vi "RW Find Edge ROI.vi"(7 "Read/Write":enum16{"Read", "Write"}(ring), 8 "error in (no error)":errorcluster, 11 "Inspec part":T1) -> (0 "error out":errorcluster)   [LabVIEW 2017]
uses:
  Use Module/Algorithm Loop/Gentex Algo/inspec part.ctl
  File/Control/Parent path.ctl
  Toolbox/Control/CVT Action.ctl
  Toolbox/Control/CVT name.vi
  Section and key name.vi
  <vilib>/Utility/config.llb/Write Key (I32).vi
  <vilib>/Utility/config.llb/Write Key (Double).vi
  <vilib>/Utility/config.llb/Read Key (I32).vi
  <vilib>/Utility/config.llb/Read Key (Double).vi
  File/File.lvlib
  <vilib>/Utility/config.llb/NI_LVConfig.lvlib
  Toolbox/Toolbox.lvlib
  Use Module/Algorithm Loop/Algorithm API.lvlib
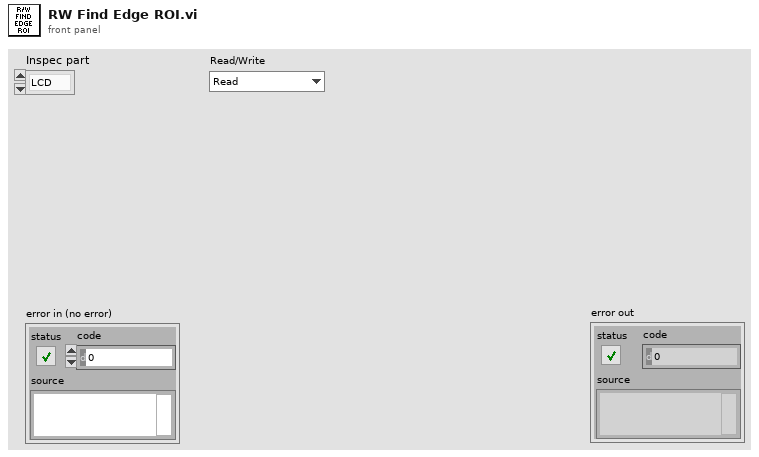
[diagram p1: front panel]
types:
  T1 = typedef "Algorithm API.lvlib/inspec part.ctl" = enum16{"LCD", "Housing"}
  T2 = typedef "File.lvlib/Parent path.ctl" = enum16{"Project", "Setting", "Log"}
  T3 = typedef "Toolbox.lvlib/CVT Action.ctl" = enum16{"Set", "Replace", "Get", "Check", "Delete", "Delete All"}
  T4 = typedef "ROI Descriptor" = cluster{"Global Rectangle":i32[], "Contours":cluster{"ID":enum32{"External", "Internal"}, "Type":u32, "Coordinates":i32[]}[]}
  T5 = typedef "IMAQ Rectangle" = cluster{"Left":i32, "Top":i32, "Right":i32, "Bottom":i32, "Rotation":dbl}
  T6 = typedef "NI_LVConfig.lvlib/Config Data RefNum.ctl" = refnum<k1>
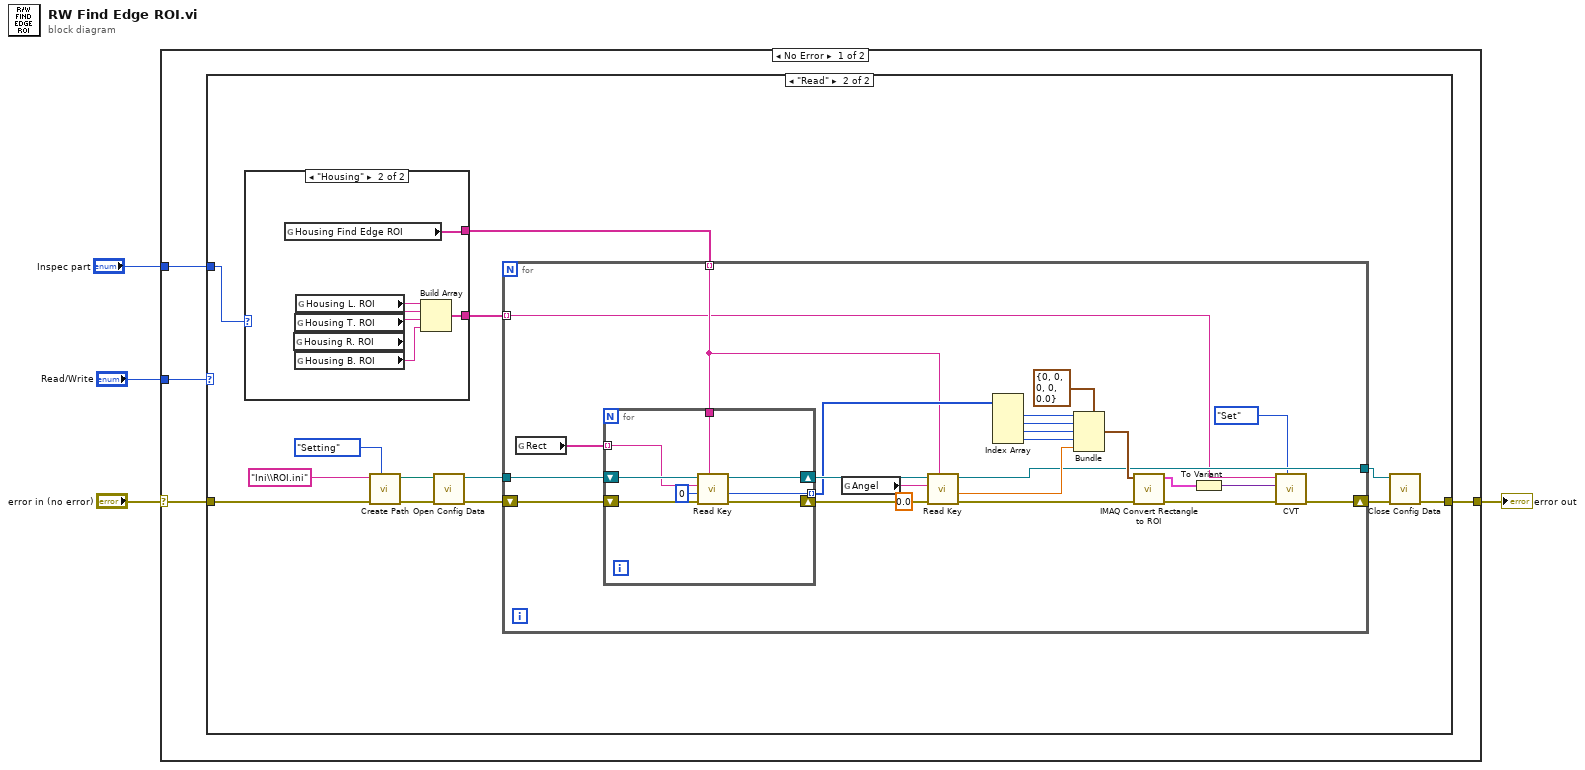
[diagram p0: block diagram]
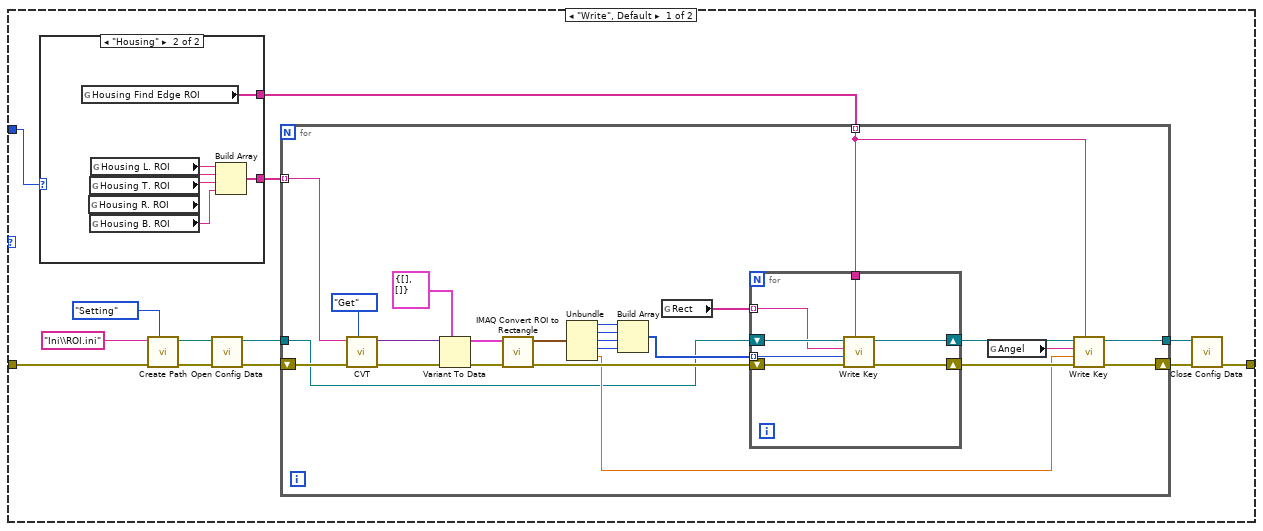
[diagram p2: hidden frame]
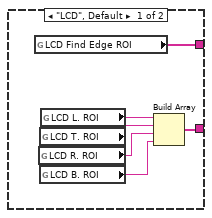
[diagram p3: hidden frame]
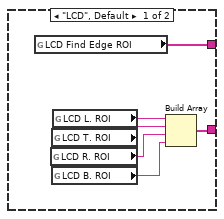
[diagram p4: hidden frame]
diagram:
  n1 = case shown="No Error" "error in (no error)" {
    selector: "error in (no error)" -> [w8 w122]
    tunnel: [w7 w122] -> w3
    tunnel: "Read/Write" -> [w6 _]
    tunnel: "Inspec part" -> [w5 _]
    frame No Error {
      n2 = case shown="\"Read\"" w6 {
        tunnel: w8 -> [w21 w77]
        tunnel: [w14 w70] -> w7
        tunnel: w5 -> [w10 w66]
        frame "Write", Default {
          n3 = case shown="\"Housing\"" w10 {
            tunnel: [w23 w29] -> w11
            tunnel: [w22 w28] -> w9
            frame "LCD", Default {
              n4 = global read "Section and key name.vi" "LCD Find Edge ROI"() -> (w22:string[])
              n5 = global read "CVT name.vi" "LCD R. ROI"() -> (w25:string)
              n6 = global read "CVT name.vi" "LCD T. ROI"() -> (w26:string)
              n7 = global read "CVT name.vi" "LCD B. ROI"() -> (w24:string)
              n8 = global read "CVT name.vi" "LCD L. ROI"() -> (w27:string)
              n9 = Build Array(w27, w26, w25, w24) -> (w23:string[])
            }
            frame "Housing" {
              n10 = global read "Section and key name.vi" "Housing Find Edge ROI"() -> (w28:string[])
              n11 = global read "CVT name.vi" "Housing R. ROI"() -> (w31:string)
              n12 = global read "CVT name.vi" "Housing T. ROI"() -> (w32:string)
              n13 = global read "CVT name.vi" "Housing B. ROI"() -> (w30:string)
              n14 = global read "CVT name.vi" "Housing L. ROI"() -> (w33:string)
              n15 = Build Array(w33, w32, w31, w30) -> (w29:string[])
            }
          }
          n16 = call "Create Path.vi"("Parent path"=Parent_path."Setting", "error in (no error)"=w21, "Directory"="Ini\\ROI.ini") -> ("error out"=w19:errorcluster, "Path"=w18:path)  [unwired: 7 in]
          n17 = call <vilib>:"Open Config Data.vi"("error in (no error)"=w19, "configuration file path"=w18) -> ("error out"=w16:errorcluster, "refnum"=w17:T6)  [unwired: 7 in, 1 out]
          n18 = for {
            tunnel: w17 -> [w35]
            shift-right: [w52] -> w15
            shift-left: w16 -> [w57]
            tunnel: [w51] -> w13
            tunnel: w11 -> [w45] mode=indexing
            tunnel: w9 -> [w34] mode=indexing
            n19 = call "CVT.vi"("Action"=CVT_Action."Get", "error in (no error)"=w57, "Key"=w45) -> ("error out"=w50:errorcluster, "Value out"=w48:variant)  [unwired: 6 in, 1 out]
            n20 = Variant To Data(error in=w50, type=T4 {"Global Rectangle"=[], "Contours"=[]} ("ROI Descriptor"), Variant=w48) -> (data=w43:T4, error out=w49:errorcluster)
            n21 = call "IMAQ Convert ROI to Rectangle"("error in (no error)"=w49, "ROI Descriptor"=w43) -> ("error out"=w44:errorcluster, "Rectangle"=w42:T5)  [unwired: 7 in]
            n22 = Unbundle(w42) -> ("Left"=w40:i32, "Top"=w39:i32, "Right"=w38:i32, "Bottom"=w37:i32, "Rotation"=w41:dbl)
            n23 = Build Array(w40, w39, w38, w37) -> (w36:i32[])
            n24 = global read "Section and key name.vi" "Rect"() -> (w54:string[])
            n25 = for {
              shift-right: [w62] -> w56
              shift-left: w35 -> [w64]
              shift-right: [w61] -> w55
              shift-left: w44 -> [w63]
              tunnel: w54 -> [w60] mode=indexing
              tunnel: w34 -> [w59]
              tunnel: w36 -> [w58] mode=indexing
              n26 = call-poly <vilib>:"Write Key.vi"("section"=w59, "error in (no error)"=w63, "value"=w58, "key"=w60, "refnum"=w64) -> ("error out"=w61:errorcluster, "refnum out"=w62:T6)  [unwired: 4 in, 1 out]
            }
            n27 = global read "Section and key name.vi" "Angel"() -> (w53:string)
            n28 = call-poly <vilib>:"Write Key.vi"("section"=w34, "error in (no error)"=w55, "value"=w41, "key"=w53, "refnum"=w56) -> ("error out"=w52:errorcluster, "refnum out"=w51:T6)  [unwired: 4 in, 1 out]
          }
          n29 = call <vilib>:"Close Config Data.vi"("error in (no error)"=w15, "refnum"=w13) -> ("error out"=w14:errorcluster)  [unwired: 8 in, 1 out]
        }
        frame "Read" {
          n30 = case shown="\"Housing\"" w66 {
            tunnel: [w79 w85] -> w68
            tunnel: [w78 w84] -> w65
            frame "LCD", Default {
              n31 = global read "Section and key name.vi" "LCD Find Edge ROI"() -> (w78:string[])
              n32 = global read "CVT name.vi" "LCD R. ROI"() -> (w81:string)
              n33 = global read "CVT name.vi" "LCD T. ROI"() -> (w82:string)
              n34 = global read "CVT name.vi" "LCD B. ROI"() -> (w80:string)
              n35 = global read "CVT name.vi" "LCD L. ROI"() -> (w83:string)
              n36 = Build Array(w83, w82, w81, w80) -> (w79:string[])
            }
            frame "Housing" {
              n37 = global read "Section and key name.vi" "Housing Find Edge ROI"() -> (w84:string[])
              n38 = global read "CVT name.vi" "Housing R. ROI"() -> (w87:string)
              n39 = global read "CVT name.vi" "Housing T. ROI"() -> (w88:string)
              n40 = global read "CVT name.vi" "Housing B. ROI"() -> (w86:string)
              n41 = global read "CVT name.vi" "Housing L. ROI"() -> (w89:string)
              n42 = Build Array(w89, w88, w87, w86) -> (w85:string[])
            }
          }
          n43 = call "Create Path.vi"("Parent path"=Parent_path."Setting", "error in (no error)"=w77, "Directory"="Ini\\ROI.ini") -> ("error out"=w75:errorcluster, "Path"=w74:path)  [unwired: 7 in]
          n44 = call <vilib>:"Open Config Data.vi"("error in (no error)"=w75, "configuration file path"=w74) -> ("error out"=w72:errorcluster, "refnum"=w73:T6)  [unwired: 7 in, 1 out]
          n45 = for {
            tunnel: w73 -> [w113]
            shift-right: [w95] -> w71
            shift-left: w72 -> [w112]
            tunnel: [w97] -> w69
            tunnel: w65 -> [w96] mode=indexing
            tunnel: w68 -> [w91] mode=indexing
            n46 = global read "Section and key name.vi" "Rect"() -> (w109:string[])
            n47 = for {
              shift-right: [w119] -> w111
              shift-left: w113 -> [w121]
              shift-right: [w118] -> w110
              shift-left: w112 -> [w120]
              tunnel: [w117] -> w106 mode=indexing
              tunnel: w109 -> [w116] mode=indexing
              tunnel: w96 -> [w115]
              n48 = call-poly <vilib>:"Read Key.vi"("section"=w115, "error in (no error)"=w120, "default value"=0, "key"=w116, "refnum"=w121) -> ("error out"=w118:errorcluster, "value"=w117:i32, "refnum out"=w119:T6)  [unwired: 3 in, 1 out]
            }
            n49 = global read "Section and key name.vi" "Angel"() -> (w108:string)
            n50 = call-poly <vilib>:"Read Key.vi"("section"=w96, "error in (no error)"=w110, "default value"=0.0, "key"=w108, "refnum"=w111) -> ("error out"=w107:errorcluster, "value"=w100:dbl, "refnum out"=w97:T6)  [unwired: 3 in, 1 out]
            n51 = Index Array(array=w106) -> (element #1=w104:i32, element #2=w103:i32, element #3=w102:i32, element #4=w101:i32)  [unwired: 4 in]
            n52 = Bundle(cluster=T5 {"Left"=0, "Top"=0, "Right"=0, "Bottom"=0, "Rotation"=0.0} ("Rectangle"), "Left"=w104, "Top"=w103, "Right"=w102, "Bottom"=w101, "Rotation"=w100) -> (w99:T5)
            n53 = call "IMAQ Convert Rectangle to ROI"("error in (no error)"=w107, "Rectangle"=w99) -> ("error out"=w98:errorcluster, "ROI Descriptor"=w94:T4)  [unwired: 7 in]
            n54 = To Variant(anything=w94) -> (Variant=w93:variant)
            n55 = call "CVT.vi"("Action"=CVT_Action."Set", "error in (no error)"=w98, "Value in"=w93, "Key"=w91) -> ("error out"=w95:errorcluster)  [unwired: 5 in, 2 out]
          }
          n56 = call <vilib>:"Close Config Data.vi"("error in (no error)"=w71, "refnum"=w69) -> ("error out"=w70:errorcluster)  [unwired: 8 in, 1 out]
        }
      }
    }
    frame Error {
    }
  }
  "error out" <- w3
